vi "Edit_Raw_DF_Header.vi"(0 "Selected files":path[](array[path])) -> ()   [LabVIEW 2021]
uses:
  Controls/File_Selector_Type.ctl
  <vilib>/Utility/error.llb/whitespace.ctl
panel:
  out "All Metadata Names":string[](array[string])
  out "New Metadata":string[](array[string])
  out "Orig Full Metadata":string[][](array[string])
  out "Meta data changed?":bool[](array[boolean])
  out "Orig Metadata Values":string[](array[string])
  out "Number of Instuments":i32
  in  "Instrument Index":i32
  in  "MetaData to change":string[][](table)
  out "Cells to Change":i32[][](array[numeric])
  out "Original Values":string[][](array[string])
  in  "Analysis Info Cluster Setup to Edit":string[][](table)
  in  "Variable names to add by hand":string[](array[string])
  in  "Variable values to add by hand":string[](array[string])
  out "No of Unfound files":i32
  out "Unfound Files":path[](array[path])
  out "File Number":i32
  out "Current case":string
  out "Currently Editting":path
  out "Summary values":string[](array[string])
  in  "New Variable values":string[](array[string])
  in  "Setup Information":i32[](listbox)
  in  "Variable names to Edit":string[](array[string])
  in  "OK":bool
  out "No of Files":i32
  in  "Previous Choice":path
  in  "Search String":string
  in  "At Dialog Prompt for Editting Raw data files":T1
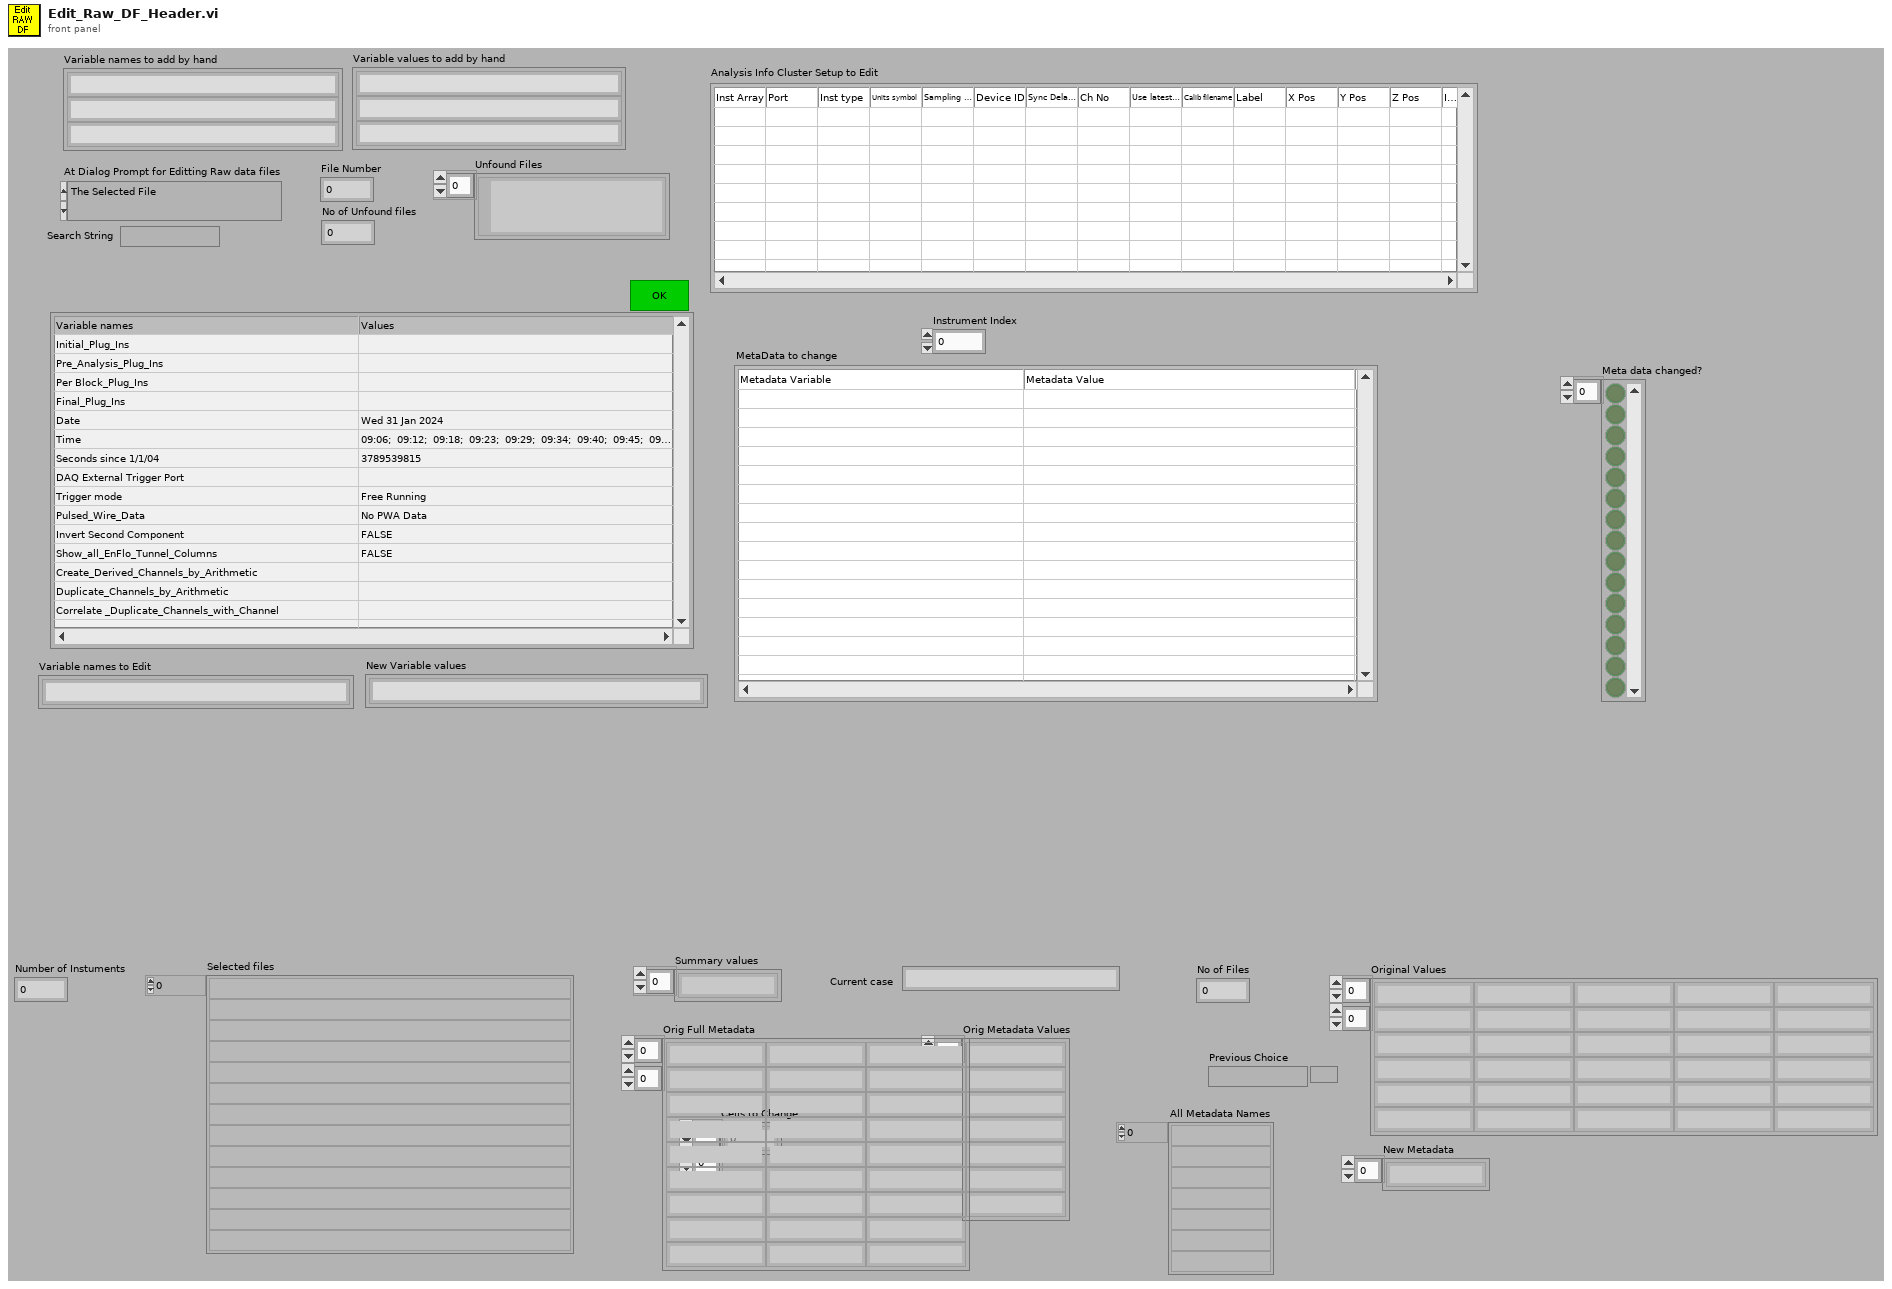
[diagram p1: front panel]
types:
  T1 = typedef "File_Selector_Type.ctl" = enum16{"The Selected File", "The Selected Folder", "Files containing the search string in the selected folder", "All files listed in selected file"}
  T2 = typedef "whitespace.ctl" = u16
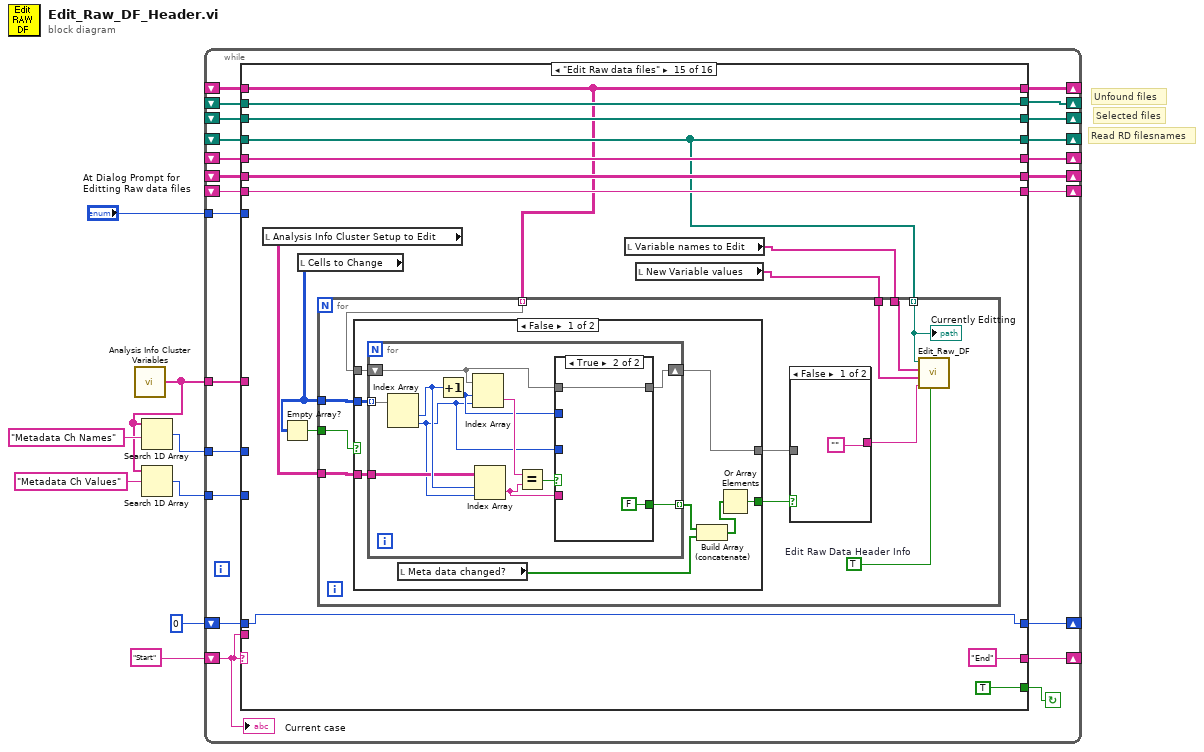
[diagram p0: block diagram]
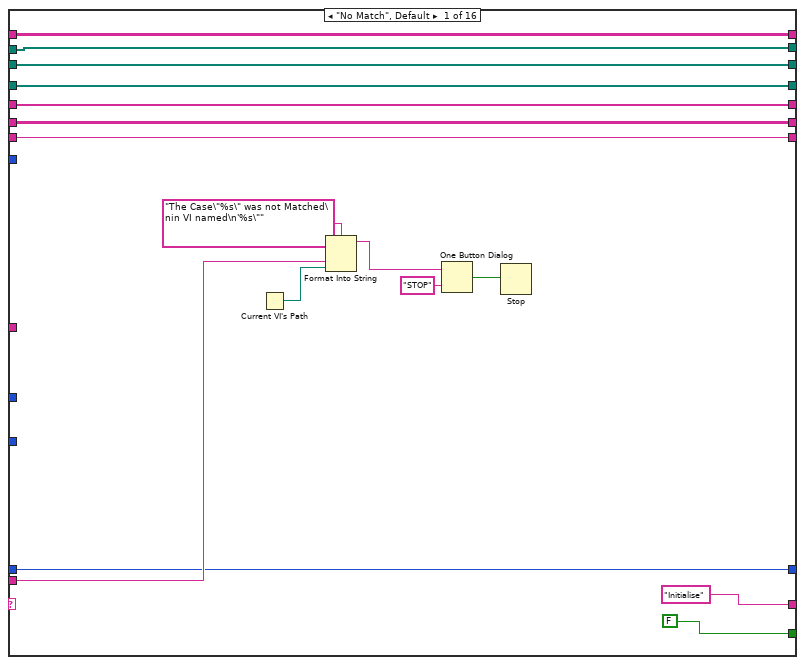
[diagram p2: hidden frame]
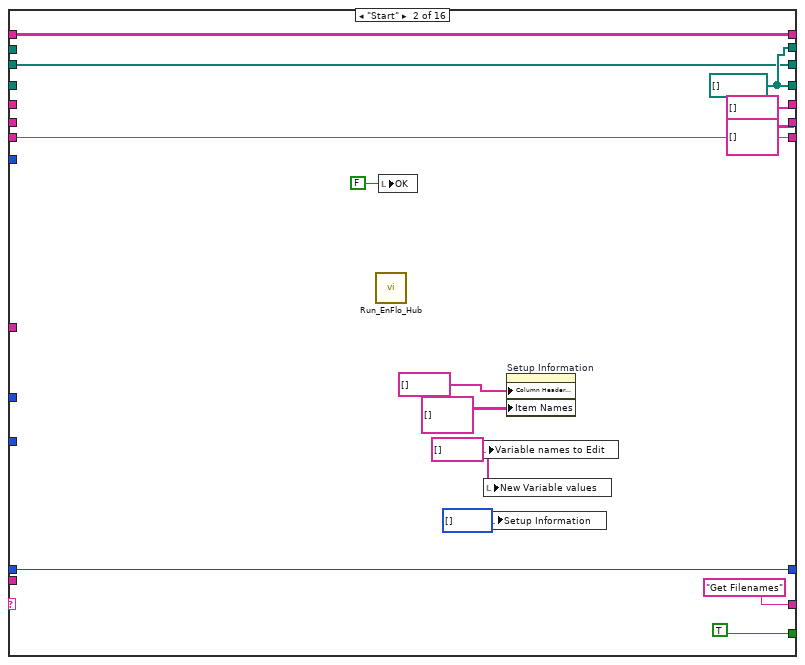
[diagram p3: hidden frame]
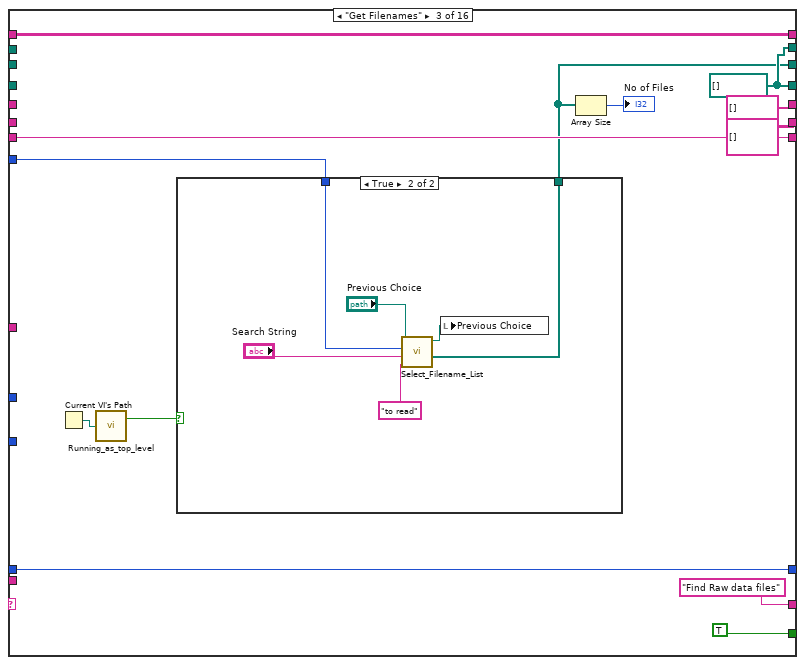
[diagram p4: hidden frame]
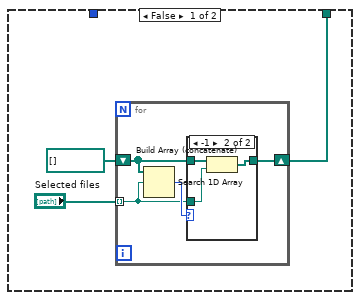
[diagram p5: hidden frame]
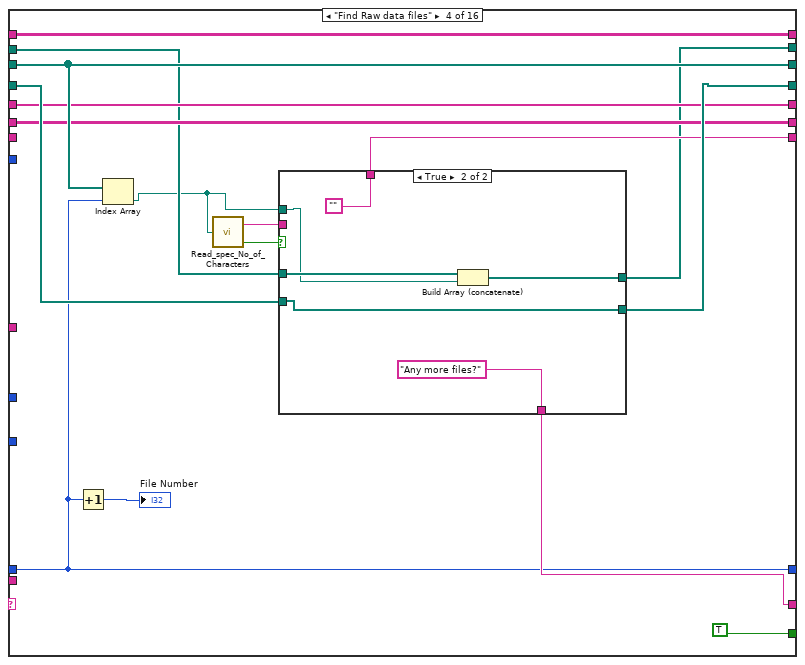
[diagram p7: hidden frame]
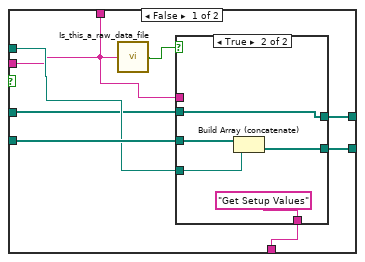
[diagram p8: hidden frame]
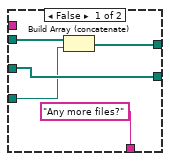
[diagram p9: hidden frame]
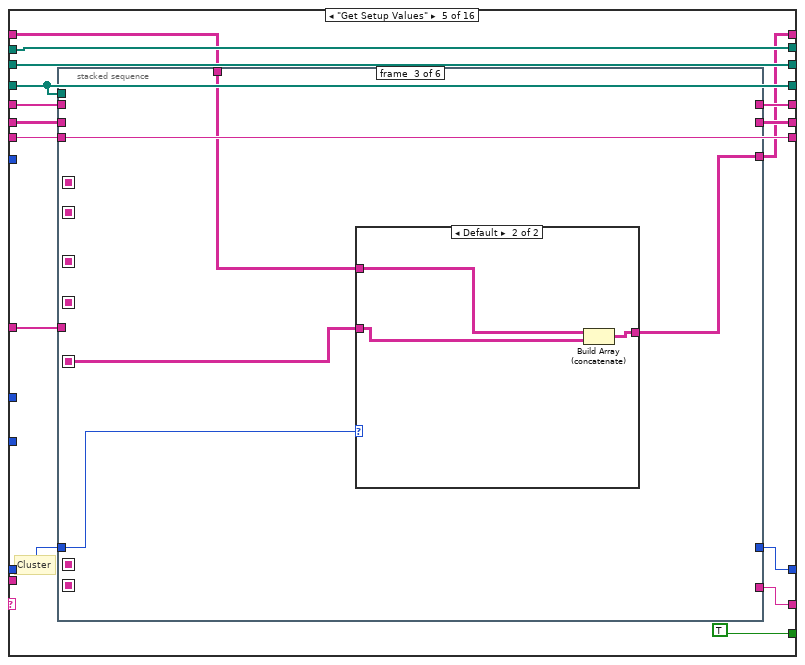
[diagram p10: hidden frame]
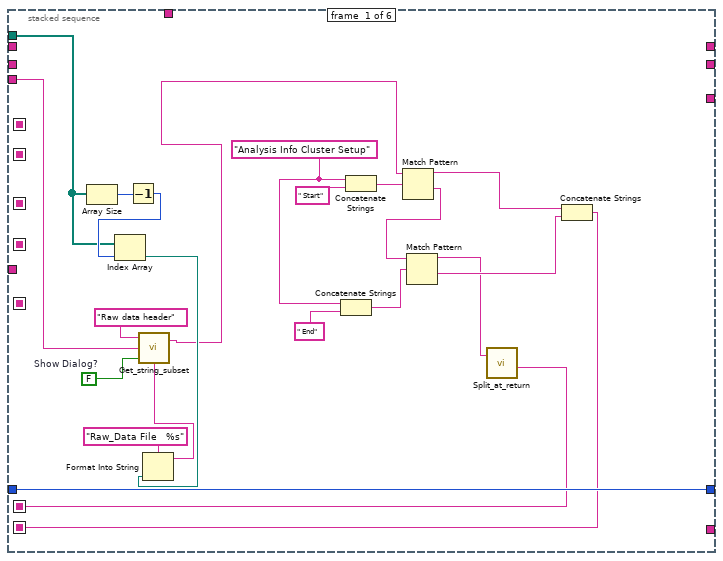
[diagram p11: hidden frame]
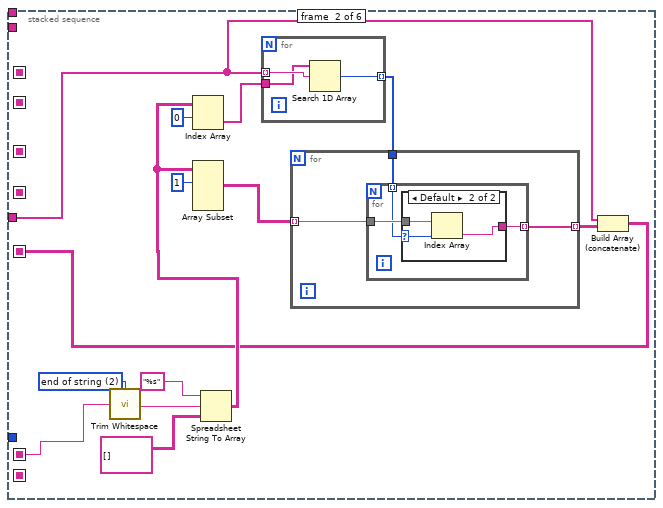
[diagram p12: hidden frame]
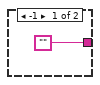
[diagram p13: hidden frame]
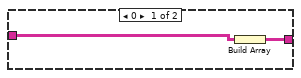
[diagram p14: hidden frame]
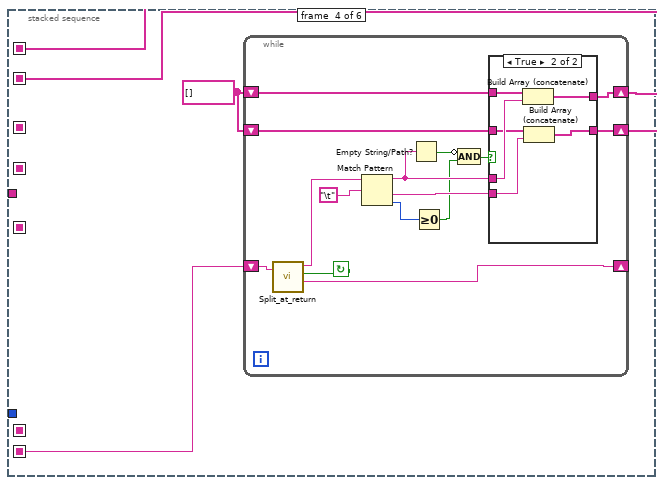
[diagram p15: hidden frame]
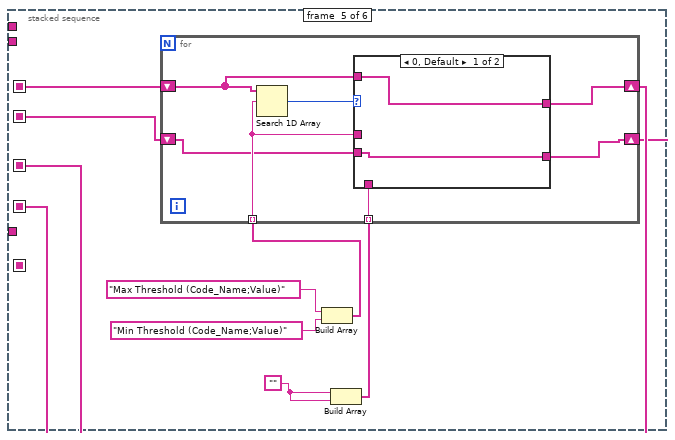
[diagram p17: hidden frame]
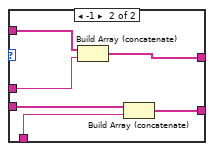
[diagram p18: hidden frame]
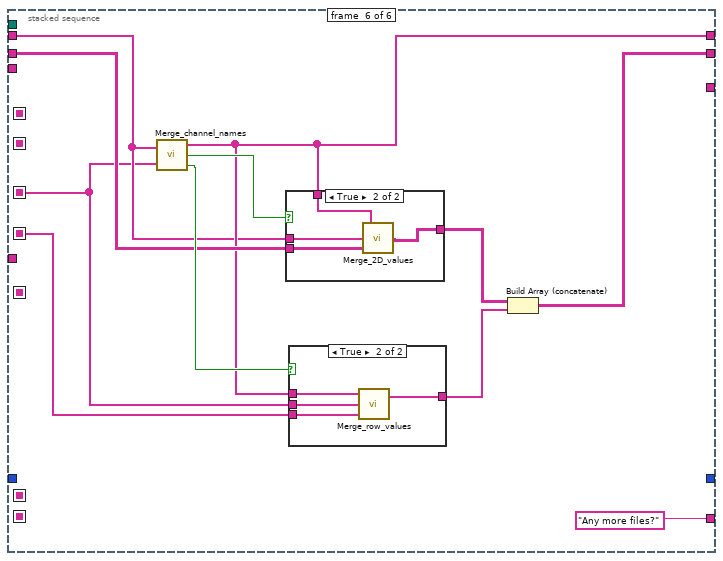
[diagram p19: hidden frame]
diagram:
  # "Selected files"
  # "Unfound files"
  # "Read RD filesnames"
  n1 = call "Analysis Info Cluster Variables.vi"() -> ("Array"=w3:string[])
  n2 = Search 1D Array(1D array=w3, element="Metadata Ch Names") -> (index of element=w1:i32)  [unwired: 1 in]
  n3 = Search 1D Array(1D array=w3, element="Metadata Ch Values") -> (index of element=w2:i32)  [unwired: 1 in]
  n4 = while {
    shift-left: "Start" -> [w29]
    shift-right: [w30] -> _
    shift-right: [w27] -> _
    shift-left: _ -> [w28]
    tunnel: "At Dialog Prompt for Editting Raw data files" -> [w26]
    shift-right: [w17] -> _
    shift-left: 0 -> [w23]
    shift-right: [w25] -> _
    shift-left: _ -> [w24]
    shift-right: [w22] -> _
    shift-left: _ -> [w21]
    shift-right: [w19] -> _
    shift-left: _ -> [w20]
    shift-right: [w18] -> _
    shift-left: _ -> [w16]
    shift-right: [w14] -> _
    shift-left: _ -> [w15]
    shift-right: [w13] -> _
    shift-left: _ -> [w12]
    tunnel: w3 -> [w11]
    tunnel: w2 -> [w10]
    tunnel: w1 -> [w9]
    stop <- w31 continue-if-true
    n5 = case shown="\"Edit Raw data files\"" w29 {
      tunnel: [FALSE TRUE TRUE TRUE TRUE TRUE TRUE TRUE TRUE TRUE ("T button?") TRUE w481 w551 TRUE ("T button?") TRUE ("T button?") FALSE ("T button?")] -> w31
      tunnel: ["Initialise" "Get Filenames" "Find Raw data files" w100 w142 w283 w303 "Summarise Analysis Cluster" "Metadata Channels" "user to select variables" w435 "Shall I edit the data files?" w544 "Edit Raw data files" ("f") "End" "End"] -> w30
      tunnel: w29 -> [w42 _ _ _ _ _ _ _ _ _ _ _ _ _ _ _]
      tunnel: w28 -> [w39 w49 _ w104 w145 w290 w309 w337 w365 w402 w441 w501 w560 w588 w634 w690]
      tunnel: [w39 w49 w63 w104 w145 w290 w309 w337 w365 w402 w441 w501 w560 w588 w634 w690] -> w27
      tunnel: w26 -> [_ _ w73 _ _ _ _ _ _ _ _ _ _ _ _ _]
      tunnel: w24 -> [w38 _ _ w106 w135 w282 w302 w334 w362 w401 w440 w498 w555 w587 w629 w684]
      tunnel: [w38 w50 w66 w105 w135 w282 w302 w334 w362 w401 w440 w498 w555 w587 w629 w684] -> w25
      tunnel: w23 -> [w34 w56 w67 w99 w144 w288 w308 w336 w364 w393 w434 w500 w556 w563 w630 w685]
      tunnel: [w37 string[] [] ("Merged Channels") string[] [] ("Merged Channels") w103 w140 w278 w297 w330 w359 w400 w436 w489 w557 w586 w631 w687] -> w22
      tunnel: w21 -> [w37 _ _ w103 w137 w278 w298 w330 w359 w400 w436 w489 w557 w586 w631 w687]
      tunnel: w20 -> [w36 _ _ w102 w139 w289 w294 w332 w360 w399 w438 w496 w558 w585 w632 w688]
      tunnel: [w36 string[][] [] string[][] [] w102 w138 w289 w293 w332 w360 w399 w438 w496 w558 w585 w632 w688] -> w19
      tunnel: [w35 w59 w70 w101 w141 w281 w301 w333 w361 w398 w439 w497 w559 w584 w633 w689] -> w18
      tunnel: [w34 w56 w67 w99 w143 w287 w307 w335 w363 w393 w434 w499 w556 w563 w630 w685] -> w17
      tunnel: w16 -> [w35 w59 w70 _ w141 w281 w301 w333 w361 w398 w439 w497 w559 w584 w633 w689]
      tunnel: w15 -> [w33 _ _ w98 w136 w279 w299 w323 w357 w403 w433 w490 w550 w583 w628 w680]
      tunnel: [w33 w50 w66 w97 w136 w279 w299 w323 w357 w403 w433 w490 w550 w583 w628 w680] -> w14
      tunnel: [w32 w48 w62 w92 w134 w277 w292 w321 w353 w396 w432 w482 w549 w565 w627 w679] -> w13
      tunnel: w12 -> [w32 w48 w62 w92 w133 w277 w292 w321 w353 w396 w432 w482 w549 w571 w627 w679]
      tunnel: w11 -> [_ _ _ _ w132 _ _ _ _ _ _ _ _ _ _ _]
      tunnel: w10 -> [_ _ _ _ _ _ _ _ _ w394 _ _ _ w567 _ _]
      tunnel: w9 -> [_ _ _ _ _ _ _ _ _ w395 _ _ _ w570 _ _]
      frame "No Match", Default {
        n6 = Current VI's Path() -> (path=w41:path)
        n7 = Format Into String(format string="The Case\"%s\" was not Matched\nin VI named\n'%s\"" ("Format String"), w42, w41) -> (resulting string=w45:string)  [unwired: 2 in, 1 out]
        n8 = One Button Dialog(message=w45, button name ("OK")="STOP") -> (true=w43:bool)
        n9 = Stop(stop? (T)=w43) -> ()
      }
      frame "Start" {
        w55 = string[] [] ("Variable names to Edit")
        w50 = path[] []
        n10 = call "Run_EnFlo_Hub.vi"() -> ()  [unwired: 1 in, 7 out]
        n11 = local write "OK"(FALSE ("OK")) -> ()
        n12 = local write "Variable names to Edit"(w55) -> ()
        n13 = local write "New Variable values"(w55) -> ()
        n14 = local write "Setup Information"(i32[] [] ("Setup Information")) -> ()
        n15 = property on="Setup Information" class="MCListbox (strict)"("Column Header Strings[]"=string[] [] ("Column Header Strings"), "Item Names"=string[][] []) -> ()  [unwired: 2 in, 2 out]
      }
      frame "Get Filenames" {
        w66 = path[] []
        n16 = Current VI's Path() -> (path=w65:path)
        n17 = call "Running_as_top_level.vi"("Vi path name"=w65) -> ("Top Level"=w64:bool)  [unwired: 1 out]
        n18 = case shown="True" w64 {
          tunnel: w73 -> [_ w91]
          tunnel: [w75 w86] -> w63
          frame False {
            n19 = for {
              shift-right: [w78] -> w75
              shift-left: path[] [] -> [w79]
              tunnel: "Selected files" -> [w80] mode=indexing
              n20 = Search 1D Array(1D array=w79, element=w80) -> (index of element=w81:i32)  [unwired: 1 in]
              n21 = case shown="-1" w81 {
                tunnel: w80 -> [_ w85]
                tunnel: w79 -> [w82 w84]
                tunnel: [w82 w83] -> w78
                frame Default {
                }
                frame -1 {
                  n22 = Build Array (concatenate)(w84, w85) -> (w83:path[])
                }
              }
            }
          }
          frame True {
            n23 = call "Select_Filename_List.vi"("File Type"="to read", "Search String"="Search String", "At Dialog Prompt Post Process"=w91, "Previous Choice"="Previous Choice") -> ("Selected files"=w86:path[], "Choosen path"=w87:path)  [unwired: 1 in, 2 out]
            n24 = local write "Previous Choice"(w87) -> ()
          }
        }
        n25 = Array Size(array=w63) -> (size(s)=→"No of Files":i32)
      }
      frame "Find Raw data files" {
        n26 = Increment(x=w99) -> (x+1=→"File Number":i32)
        n27 = Index Array(array=w104, index=w99) -> (element=w96:path)
        n28 = call "Read_spec_No_of_Characters.vi"("Filename"=w96) -> ("character string"=w94:string, "Error?"=w95:bool)
        n29 = case shown="True" w95 {
          tunnel: w106 -> [w115 w131]
          tunnel: [w114 w131] -> w105
          tunnel: w96 -> [w112 w127]
          tunnel: [w108 ""] -> w101
          tunnel: [w111 "Any more files?"] -> w100
          tunnel: w98 -> [w110 w128]
          tunnel: [w109 w126] -> w97
          tunnel: w94 -> [w108 _]
          frame False {
            n30 = call "Is_this_a_raw_data_file.vi"("character string"=w108) -> ("Raw Dat File?"=w113:bool)  [unwired: 2 out]
            n31 = case shown="True" w113 {
              tunnel: w115 -> [w120 w125]
              tunnel: w112 -> [w116 w124]
              tunnel: [w120 w123] -> w114
              tunnel: w108 -> [_ _]
              tunnel: ["Any more files?" "Get Setup Values"] -> w111
              tunnel: w110 -> [w118 w121]
              tunnel: [w117 w121] -> w109
              frame False {
                n32 = Build Array (concatenate)(w118, w116) -> (w117:path[])
              }
              frame True {
                n33 = Build Array (concatenate)(w125, w124) -> (w123:path[])
              }
            }
          }
          frame True {
            n34 = Build Array (concatenate)(w128, w127) -> (w126:path[])
          }
        }
      }
      frame "Get Setup Values" {
        # "Cluster"
        n35 = stacked-sequence {
          seq-local: [_ _ _ w207 _ _] -> [_ _ _ _ w240 _]
          seq-local: [_ _ _ w206 _ _] -> [_ _ _ _ w236 _]
          seq-local: [_ _ _ _ w233 _] -> [_ _ _ _ _ w257]
          seq-local: [_ _ _ _ w232 _] -> [_ _ _ _ _ w256]
          seq-local: [w149 _ _ _ _ _] -> [_ _ _ w205 _ _]
          seq-local: [w147 _ _ _ _ _] -> [_ w170 _ _ _ _]
          seq-local: [_ w172 _ _ _ _] -> [_ _ w196 _ _ _]
          tunnel: w144 -> [w165 _ w199 _ _ _]
          tunnel: [w165 _ _ _ _ _] -> w143
          tunnel: [_ _ _ _ _ "Any more files?"] -> w142
          tunnel: w141 -> [w166 _ _ _ _ _]
          tunnel: w137 -> [_ _ _ _ _ w258]
          tunnel: [_ _ _ _ _ w260] -> w140
          tunnel: w139 -> [_ _ _ _ _ w264]
          tunnel: [_ _ _ _ _ w261] -> w138
          tunnel: w135 -> [w160 _ _ _ _ _]
          tunnel: [_ _ w198 _ _ _] -> w134
          tunnel: w133 -> [_ _ w197 _ _ _]
          tunnel: w132 -> [_ w173 _ _ _ _]
          frame #0 {
            w155 = "Analysis Info Cluster Setup"
            w168 = FALSE  # Show Dialog?
            n36 = Array Size(array=w160) -> (size(s)=w162:i32)
            n37 = Decrement(x=w162) -> (x-1=w161:i32)
            n38 = Index Array(array=w160, index=w161) -> (element=w159:path)
            n39 = Format Into String(format string="Raw_Data File   %s", w159) -> (resulting string=w163:string)  [unwired: 2 in, 1 out]
            n40 = call "Get_string_subset.vi"("String Name"=w163, "Show Dialog?"=w168, "String to split"=w166, "File Label"="Raw data header") -> ("Output string"=w154:string)  [unwired: 1 out]
            n41 = Concatenate Strings(w155, " End") -> (w152:string)
            n42 = Concatenate Strings(w155, " Start") -> (w158:string)
            n43 = Match Pattern(string=w154, regular expression=w158) -> (before substring=w151:string, after substring=w153:string)  [unwired: 3 out]
            n44 = Match Pattern(string=w153, regular expression=w152) -> (before substring=w148:string, after substring=w150:string)  [unwired: 3 out]
            n45 = call "Split_at_return.vi"("String"=w148) -> ("after substring"=w147:string)  [unwired: 1 in, 3 out]
            n46 = Concatenate Strings(w151, w150) -> (w149:string)
          }
          frame #1 {
            w171 = T2 2 items=["both", "start of string", "end of string"] ("location (both)")
            n47 = call <vilib>:"Trim Whitespace.vi"("string"=w170, "location (both)"=w171) -> ("trimmed string"=w169:string)
            n48 = Spreadsheet String To Array(format string="%s", spreadsheet string=w169, array type (2D Dbl)=string[][] []) -> (array=w178:string[][])  [unwired: 1 in]
            n49 = Index Array(array=w178, index (row)=0) -> (element=w179:string[])  [unwired: 1 in]
            n50 = Array Subset(array=w178, index (row)=1 ("index")) -> (w176:string[][])  [unwired: 3 in]
            n51 = for {
              tunnel: w173 -> [w195] mode=indexing
              tunnel: w179 -> [w194]
              tunnel: [w193] -> w175 mode=indexing
              n52 = Search 1D Array(1D array=w194, element=w195) -> (index of element=w193:i32)  [unwired: 1 in]
            }
            n53 = for {
              tunnel: w176 -> [w185] mode=indexing
              tunnel: w175 -> [w184]
              tunnel: [w183] -> w174 mode=indexing
              n54 = for {
                tunnel: w185 -> [w188]
                tunnel: w184 -> [w187] mode=indexing
                tunnel: [w186] -> w183 mode=indexing
                n55 = case shown="Default" w187 {
                  selector: w187 -> [_ w191]
                  tunnel: w188 -> [_ w192]
                  tunnel: ["" w190] -> w186
                  frame -1 {
                  }
                  frame Default {
                    n56 = Index Array(array=w192, index=w191) -> (element=w190:string)
                  }
                }
              }
            }
            n57 = Build Array (concatenate)(w173, w174) -> (w172:string[][])
          }
          frame #2 {
            n58 = case shown="Default" w199 {
              tunnel: w196 -> [w201 w203]
              tunnel: [w200 w202] -> w198
              tunnel: w197 -> [_ w204]
              frame 0 {
                n59 = Build Array(w201) -> (w200:string[][][])
              }
              frame Default {
                n60 = Build Array (concatenate)(w204, w203) -> (w202:string[][][])
              }
            }
          }
          frame #3 {
            w208 = string[] []
            n61 = while {
              shift-right: [w222] -> _
              shift-left: w205 -> [w223]
              shift-right: [w216] -> w207
              shift-left: w208 -> [w217]
              shift-right: [w214] -> w206
              shift-left: w208 -> [w215]
              stop <- w221 continue-if-true
              n62 = call "Split_at_return.vi"("String"=w223) -> ("before substring"=w219:string, "Matched?"=w221:bool, "after substring"=w222:string)  [unwired: 1 in, 1 out]
              n63 = Match Pattern(string=w219, regular expression="\t") -> (before substring=w212:string, after substring=w213:string, offset past match=w218:i32)  [unwired: 2 out]
              n64 = Empty String/Path?(string/path=w212) -> (empty?=w211:bool)
              n65 = Greater Or Equal To 0?(x=w218) -> (x >= 0?=w209:bool)
              n66 = Compound Arithmetic op=AND(invert w211, w209) -> (w210:bool)
              n67 = case shown="True" w210 {
                tunnel: w217 -> [w225 w231]
                tunnel: w212 -> [_ w230]
                tunnel: [w225 w229] -> w216
                tunnel: w215 -> [w224 w228]
                tunnel: [w224 w227] -> w214
                tunnel: w213 -> [_ w226]
                frame False {
                }
                frame True {
                  n68 = Build Array (concatenate)(w231, w230) -> (w229:string[])
                  n69 = Build Array (concatenate)(w228, w226) -> (w227:string[])
                }
              }
            }
          }
          frame #4 {
            w234 = ""
            n70 = Build Array("Max Threshold (Code_Name;Value)", "Min Threshold (Code_Name;Value)") -> (w237:string[])
            n71 = Build Array(w234, w234) -> (w235:string[])
            n72 = for {
              shift-right: [w244] -> w233
              shift-left: w240 -> [w246]
              tunnel: w237 -> [w245] mode=indexing
              shift-right: [w241] -> w232
              shift-left: w236 -> [w243]
              tunnel: w235 -> [w242] mode=indexing
              n73 = Search 1D Array(1D array=w246, element=w245) -> (index of element=w247:i32)  [unwired: 1 in]
              n74 = case shown="0, Default" w247 {
                tunnel: w246 -> [w249 w255]
                tunnel: w245 -> [_ w254]
                tunnel: [w249 w253] -> w244
                tunnel: w243 -> [w248 w252]
                tunnel: w242 -> [_ w251]
                tunnel: [w248 w250] -> w241
                frame 0, Default {
                }
                frame -1 {
                  n75 = Build Array (concatenate)(w255, w254) -> (w253:string[])
                  n76 = Build Array (concatenate)(w252, w251) -> (w250:string[])
                }
              }
            }
          }
          frame #5 {
            n77 = call "Merge_channel_names.vi"("Preferred Channel array"=w258, "Channel array"=w257) -> ("Merged Channels"=w260:string[], "Preferred Channels Changed?"=w265:bool, "Channel Array Changed?"=w266:bool)
            n78 = case shown="True" w265 {
              tunnel: w264 -> [w272 w274]
              tunnel: w258 -> [_ w276]
              tunnel: [w272 w273] -> w263
              tunnel: w260 -> [_ w275]
              frame False {
              }
              frame True {
                n79 = call "Merge_2D_values.vi"("Values In"=w274, "Present Channels"=w276, "Desired Channels"=w275) -> ("Values Out"=w273:string[][])
              }
            }
            n80 = case shown="True" w266 {
              tunnel: [w267 w271] -> w262
              tunnel: w260 -> [_ w270]
              tunnel: w257 -> [_ w269]
              tunnel: w256 -> [w267 w268]
              frame False {
              }
              frame True {
                n81 = call "Merge_row_values.vi"("Present Row values"=w268, "Present Channels"=w269, "Desired Channels"=w270) -> ("Desired Row values"=w271:string[])  [unwired: 1 out]
              }
            }
            n82 = Build Array (concatenate)(w263, w262) -> (w261:string[][])
          }
        }
      }
      frame "Any more files?" {
        n83 = Increment(x=w288) -> (x+1=w287:i32)
        n84 = local read "No of Files"() -> (w286:i32)
        n85 = Less?(x=w287, y=w286) -> (x < y?=w285:bool)
        n86 = Select(t="Find Raw data files", s=w285, f="Add Skip Blocks Variable") -> (s? t:f=w283:string)
      }
      frame "Add Skip Blocks Variable" {
        w296 = "Skip_Block_Numbers_(eg 1;2;5;12)" ("Variable name")
        n87 = Increment(x=w308) -> (x+1=w307:i32)
        n88 = Search 1D Array(1D array=w298, element=w296) -> (index of element=w295:i32)  [unwired: 1 out]
        n89 = case shown="-1" w295 {
          tunnel: w298 -> [w312 w317]
          tunnel: w296 -> [_ w316]
          tunnel: [w312 w315] -> w297
          tunnel: w294 -> [w311 w314]
          tunnel: [w311 w313] -> w293
          frame 0, Default {
          }
          frame -1 {
            n90 = for {
              tunnel: w314 -> [w319] mode=indexing
              tunnel: [w318] -> w313 mode=indexing
              n91 = Build Array (concatenate)(w319, "") -> (w318:string[])
            }
            n92 = Build Array (concatenate)(w317, w316) -> (w315:string[])
          }
        }
        n93 = local read "No of Files"() -> (w306:i32)
        n94 = Less?(x=w307, y=w306) -> (x < y?=w305:bool)
        n95 = Select(t="Find Raw data files", s=w305, f="Summarise data") -> (s? t:f=w303:string)
      }
      frame "Summarise data" {
        n96 = Increment(x=w336) -> (x+1=w335:i32)
        n97 = Array Size(array=w330) -> (size(s)=w331:i32)
        n98 = for {
          N: w331 -> [_]
          tunnel: w332 -> [w346]
          tunnel: [w342] -> w329 mode=indexing
          i -> [w347]
          w343 = FALSE  # Average Numeric Values?
          n99 = Index Array(array=w346, index (col)=w347) -> (element=w345:string[])  [unwired: 1 in]
          n100 = call "Value_Occurence_Analysis.vi"("Average Numeric Values?"=w343, "Tolerance"=0.5, "String Array"=w345) -> ("Output String"=w342:string)  [unwired: 1 in, 2 out]
        }
        "Summary values" <- w329
        n101 = for {
          tunnel: w330 -> [w340] mode=indexing
          tunnel: w329 -> [w341] mode=indexing
          tunnel: [w339] -> w325 mode=indexing
          n102 = Build Array(w340, w341) -> (w339:string[])
        }
        n103 = Array Size(array=w323) -> (size(s)=→"No of Unfound files":i32)
        n104 = Build Array("Variable names", "Values") -> (w324:string[])
        n105 = property on="Setup Information" class="MCListbox (strict)"("Column Header Strings[]"=w324, "Item Names"=w325) -> ()  [unwired: 2 in, 2 out]
        "Unfound Files" <- w323
      }
      frame "Summarise Analysis Cluster" {
        n106 = Array Size(array=w353) -> (size(s)=w356:i32[])
        n107 = Index Array(array=w356) -> (element #2=w355:i32, element #3=w354:i32)  [unwired: 3 in, 1 out]
        "Number of Instuments" <- w355
        n108 = Increment(x=w364) -> (x+1=w363:i32)
        n109 = for {
          N: w355 -> [_]
          tunnel: w353 -> [w369]
          tunnel: [w370] -> w351 mode=indexing
          tunnel: w354 -> [w367]
          i -> [w368]
          n110 = for {
            N: w367 -> [_]
            tunnel: [w372] -> w370 mode=indexing
            tunnel: w369 -> [w375]
            tunnel: w368 -> [w374]
            i -> [w373]
            n111 = Index Array(array=w375, index (dim 1)=w374, index (dim 2)=w373) -> (element=w371:string[])  [unwired: 1 in]
            n112 = call "Value_Occurence_Analysis.vi"("Average Numeric Values?"=FALSE, "Tolerance"=0.5, "String Array"=w371) -> ("Output String"=w372:string)  [unwired: 1 in, 2 out]
          }
        }
        n113 = Array Subset(array=w351, index (row)=1 ("index")) -> (w349:string[][])  [unwired: 3 in]
        "Original Values" <- w349
        n114 = local write "Analysis Info Cluster Setup to Edit"(w349) -> ()
        n115 = Index Array(array=w351, index (row)=0) -> (element=w348:string[])  [unwired: 1 in]
        n116 = property on="Analysis Info Cluster Setup to Edit" class="Tbl (strict)"("Column Headers[]"=w348) -> ()  [unwired: 2 in, 2 out]
      }
      frame "Metadata Channels" {
        n117 = local read "Number of Instuments"() -> (w383:i32)
        n118 = Array Subset(array=w396, index (dim 1)=1 ("index")) -> (w390:string[][][])  [unwired: 5 in]
        n119 = Greater?(x=w383, y="Instrument Index") -> (0:w382:bool)
        n120 = case shown="False" w382 {
          tunnel: [w404 w405] -> w381
          tunnel: "Instrument Index" -> [w404 _]
          frame False {
          }
          frame True {
            w405 = 0 ("Instrument Index")
            n121 = local write "Instrument Index"(w405) -> ()
          }
        }
        n122 = Index Array(array=w390, index (dim 1)=w381, index (dim 2)=w395) -> (element=w388:string[])  [unwired: 1 in]
        n123 = Index Array(array=w390, index (dim 1)=w381, index (dim 2)=w394) -> (element=w387:string[])  [unwired: 1 in]
        n124 = for {
          tunnel: w388 -> [w430] mode=indexing
          tunnel: [w429] -> w389 mode=concatenating
          n125 = call "String_2_String_Array.vi"("delimiter (;)"=";", "String"=w430) -> ("String Array"=w429:string[])  [unwired: 9 in]
        }
        n126 = call "Analyse_string_array.vi"("String array"=w389) -> ("Unique strings"=w385:string[])  [unwired: 1 in, 1 out]
        "All Metadata Names" <- w385
        n127 = for {
          tunnel: w388 -> [w418] mode=indexing
          tunnel: w387 -> [w416] mode=indexing
          tunnel: w385 -> [w415]
          tunnel: [w412] -> w386 mode=indexing
          n128 = call "String_2_String_Array.vi"("delimiter (;)"=";", "String"=w416) -> ("String Array"=w413:string[])  [unwired: 9 in]
          n129 = call "String_2_String_Array.vi"("delimiter (;)"=";", "String"=w418) -> ("String Array"=w414:string[])  [unwired: 9 in]
          n130 = for {
            tunnel: w415 -> [w424] mode=indexing
            tunnel: w414 -> [w423]
            tunnel: w413 -> [w421]
            tunnel: [w420] -> w412 mode=indexing
            n131 = Search 1D Array(1D array=w423, element=w424) -> (index of element=w422:i32)  [unwired: 1 in]
            n132 = case shown="-1" w422 {
              selector: w422 -> [w426 _]
              tunnel: w421 -> [w427 _]
              tunnel: [w425 ""] -> w420
              frame 0, Default {
                n133 = Index Array(array=w427, index=w426) -> (element=w425:string)
              }
              frame -1 {
              }
            }
          }
        }
        n134 = Transpose 2D Array(2D array=w386) -> (transposed array=w378:string[][])
        "Orig Full Metadata" <- w378
        n135 = for {
          tunnel: w378 -> [w409] mode=indexing
          tunnel: w385 -> [w408] mode=indexing
          tunnel: [w407] -> w384 mode=indexing
          tunnel: [w406] -> w379 mode=indexing
          n136 = call "Value_Occurence_Analysis.vi"("Average Numeric Values?"=FALSE, "Tolerance"=0.5, "String Array"=w409) -> ("Output String"=w406:string)  [unwired: 1 in, 2 out]
          n137 = Build Array(w408, w406) -> (w407:string[])
        }
        "Orig Metadata Values" <- w379
        n138 = local write "MetaData to change"(w384) -> ()
      }
      frame "user to select variables" {
        n139 = event shown="[0] \"Setup Information\": Value Change" {
          selector: _ -> [_ _]
          dyn-events: _ -> [_ _]
          timeout: _ -> [_ _]
          tunnel: w436 -> [w450 _]
          tunnel: ["user to select variables" "Any files to edit?"] -> w435
          event "Setup Information": Value Change {
            n140 = event-data() -> ("NewVal"=w451:i32[])  [unwired: 6 out]
            n141 = local read "Summary values"() -> (w449:string[])
            n142 = for {
              tunnel: w451 -> [w457] mode=indexing
              tunnel: w450 -> [w460]
              tunnel: "Variable names to Edit" -> [w459]
              tunnel: [w458] -> w443 mode=indexing
              tunnel: w449 -> [w456]
              tunnel: [w455] -> w448 mode=indexing
              tunnel: "New Variable values" -> [w453]
              tunnel: [w452] -> w445
              i -> [w452]
              n143 = Index Array(array=w460, index=w457) -> (element=w458:string)
              n144 = Search 1D Array(1D array=w459, element=w458) -> (index of element=w454:i32)  [unwired: 1 out]
              n145 = case shown="-1" w454 {
                tunnel: w457 -> [_ w466]
                tunnel: w456 -> [_ w465]
                tunnel: [w461 w464] -> w455
                tunnel: w454 -> [w463 _]
                tunnel: w453 -> [w462 _]
                frame 0, Default {
                  n146 = Index Array(array=w462, index=w463) -> (element=w461:string)
                }
                frame -1 {
                  n147 = Index Array(array=w465, index=w466) -> (element=w464:string)
                }
              }
            }
            n148 = Increment(x=w445) -> (x+1=w444:i32)
            n149 = local write "New Variable values"(w448) -> ()
            n150 = local write "Variable names to Edit"(w443) -> ()
            n151 = property on="Variable names to Edit" class="Arr (strict)"("Number of Rows"=w444) -> ()  [unwired: 2 in, 2 out]
            n152 = property on="New Variable values" class="Arr (strict)"("Number of Rows"=w444) -> ()  [unwired: 2 in, 2 out]
          }
          event "OK": Value Change {
            n153 = event-data() -> ()  [unwired: 7 out]
          }
        }
      }
      frame "Any files to edit?" {
        w492 = string[] []
        n154 = local read "New Variable values"() -> (w488:string[])
        n155 = Increment(x=w500) -> (x+1=w499:i32)
        n156 = local read "Summary values"() -> (w493:string[])
        n157 = local read "Original Values"() -> (w479:string[][])
        n158 = local read "Variable names to Edit"() -> (w485:string[])
        n159 = Build Array (concatenate)("Variable values to add by hand", w488) -> (w486:string[])
        n160 = for {
          tunnel: "Analysis Info Cluster Setup to Edit" -> [w506] mode=indexing
          tunnel: w479 -> [w505] mode=indexing
          shift-right: [w502] -> w477
          shift-left: i32[][] [] -> [w503]
          i -> [w504]
          n161 = for {
            tunnel: w506 -> [w513] mode=indexing
            tunnel: w505 -> [w512] mode=indexing
            tunnel: w504 -> [w511]
            shift-right: [w508] -> w502
            shift-left: w503 -> [w507]
            i -> [w510]
            n162 = Equal?(x=w513, y=w512) -> (x = y?=w509:bool)
            n163 = case shown="False" w509 {
              tunnel: w511 -> [w518 _]
              tunnel: w510 -> [w517 _]
              tunnel: [w515 w519] -> w508
              tunnel: w507 -> [w514 w519]
              frame False {
                n164 = Build Array(w518, w517) -> (w516:i32[])
                n165 = Build Array (concatenate)(w516, w514) -> (w515:i32[][])
              }
              frame True {
              }
            }
          }
        }
        "Cells to Change" <- w477
        n166 = Build Array (concatenate)("Variable names to add by hand", w485) -> (w483:string[])
        n167 = for {
          tunnel: "Setup Information" -> [w522]
          tunnel: w493 -> [w535]
          tunnel: w486 -> [w529] mode=indexing
          shift-right: [w532] -> w491
          shift-left: w492 -> [w533]
          shift-right: [w530] -> w475
          shift-left: w492 -> [w531]
          tunnel: w483 -> [w527] mode=indexing
          tunnel: w489 -> [w528]
          i -> [w521]
          n168 = Index Array(array=w522, index=w521) -> (element=w520:i32)
          n169 = Index Array(array=w528, index=w520) -> (element=w526:string)
          n170 = Index Array(array=w535, index=w520) -> (element=w534:string)
          n171 = Equal?(x=w534, y=w529) -> (x = y?=w525:bool)
          n172 = Equal?(x=w527, y=w526) -> (x = y?=w524:bool)
          n173 = And(x=w524, y=w525) -> (x .and. y?=w523:bool)
          n174 = case shown="False" w523 {
            tunnel: w533 -> [w541 w543]
            tunnel: [w540 w543] -> w532
            tunnel: w531 -> [w539 w542]
            tunnel: [w538 w542] -> w530
            tunnel: w529 -> [w537 _]
            tunnel: w527 -> [w536 _]
            frame False {
              n175 = Build Array (concatenate)(w539, w537) -> (w538:string[])
              n176 = Build Array (concatenate)(w541, w536) -> (w540:string[])
            }
            frame True {
            }
          }
        }
        n177 = local write "Variable names to Edit"(w491) -> ()
        n178 = local read "Orig Metadata Values"() -> (w470:string[])
        n179 = Empty Array?(array=w477) -> (empty?=w476:bool)
        n180 = Index Array(array="MetaData to change", index (col)=1 ("disabled index (col)")) -> (element=w471:string[])  [unwired: 1 in]
        "New Metadata" <- w471
        n181 = local write "New Variable values"(w475) -> ()
        n182 = Empty Array?(array=w475) -> (empty?=w474:bool)
        n183 = Not Equal?(x=w471, y=w470) -> (x != y?=w469:bool[])
        "Meta data changed?" <- w469
        n184 = Or Array Elements(Boolean array=w469) -> (logical OR=w468:bool)
        n185 = Compound Arithmetic op=OR(w468, invert w474, invert w476) -> (w481:bool)
      }
      frame "Shall I edit the data files?" {
        n186 = Array Size(array=w555) -> (size(s)=w554:i32)
        n187 = local read "Meta data changed?"() -> (w548:bool[])
        n188 = Format Into String(format string="Do you want to edit these raw data header values in %d Raw Data Files?" ("message"), w554) -> (resulting string=w552:string)  [unwired: 2 in, 1 out]
        n189 = Or Array Elements(Boolean array=w548) -> (logical OR=w547:bool)
        n190 = Two Button Dialog(message=w552) -> (T button?=w551:bool)  [unwired: 2 out]
        n191 = Select(t="Update metadata", s=w547, f="Edit Raw data files") -> (s? t:f=w544:string)
        n192 = property on="Currently Editting" class="Path"("Visible"=w551) -> ()  [unwired: 2 in, 2 out]
      }
      frame "Update metadata" {
        n193 = local read "Orig Full Metadata"() -> (w581:string[][])
        n194 = local read "Instrument Index"() -> (w569:i32)
        n195 = local read "Meta data changed?"() -> (w582:bool[])
        n196 = local read "All Metadata Names"() -> (w576:string[])
        n197 = local read "New Metadata"() -> (w578:string[])
        n198 = Array Size(array=w581) -> (size(s)=w580:i32[])
        n199 = Increment(x=w569) -> (x+1=w561:i32)
        n200 = Index Array(array=w580, index=1) -> (element=w579:i32)
        n201 = for {
          tunnel: w582 -> [w615] mode=indexing
          tunnel: [w614] -> w577 mode=indexing
          tunnel: w581 -> [w613] mode=indexing
          tunnel: w579 -> [w612]
          tunnel: w578 -> [w611] mode=indexing
          n202 = case shown="True" w615 {
            tunnel: [w616 w617] -> w614
            tunnel: w613 -> [w616 _]
            tunnel: w612 -> [_ w619]
            tunnel: w611 -> [_ w618]
            frame False {
            }
            frame True {
              n203 = Initialize Array(w618, w619) -> (w617:string[])
            }
          }
        }
        n204 = for {
          shift-right: [w607] -> w568
          shift-left: "" -> [w610]
          tunnel: ";" ("delimiter (Tab)") -> [w609]
          tunnel: w576 -> [w606] mode=indexing
          n205 = call <vilib>:"Space Constant.vi"() -> ("String"=w608:string)
          n206 = Concatenate Strings(w610, w606, w609, w608) -> (w607:string)
        }
        n207 = Transpose 2D Array(2D array=w577) -> (transposed array=w575:string[][])
        n208 = for {
          tunnel: w575 -> [w598] mode=indexing
          tunnel: [w597] -> w566 mode=indexing
          n209 = for {
            shift-right: [w602] -> w597
            shift-left: "" -> [w605]
            tunnel: ";" ("delimiter (Tab)") -> [w604]
            tunnel: w598 -> [w601] mode=indexing
            n210 = call <vilib>:"Space Constant.vi"() -> ("String"=w603:string)
            n211 = Concatenate Strings(w605, w601, w604, w603) -> (w602:string)
          }
        }
        n212 = for {
          tunnel: w571 -> [w594] mode=indexing
          tunnel: w570 -> [w590]
          tunnel: w561 -> [w591]
          tunnel: w568 -> [w596]
          tunnel: w567 -> [w589]
          tunnel: w566 -> [w595] mode=indexing
          tunnel: [w593] -> w565 mode=indexing
          n213 = Replace Array Subset(array=w594, new element=w596, index (row)=w591, index (col)=w590) -> (w592:string[][])
          n214 = Replace Array Subset(array=w592, new element=w595, index (row)=w591, index (col)=w589) -> (w593:string[][])
        }
      }
      frame "Edit Raw data files" {
        n215 = local read "Analysis Info Cluster Setup to Edit"() -> (w626:string[][])
        n216 = local read "Cells to Change"() -> (w621:i32[][])
        n217 = Empty Array?(array=w621) -> (empty?=w620:bool)
        n218 = local read "Variable names to Edit"() -> (w625:string[])
        n219 = local read "New Variable values"() -> (w624:string[])
        n220 = for {
          tunnel: w627 -> [w644] mode=indexing
          tunnel: w621 -> [w636]
          tunnel: w626 -> [w645]
          tunnel: w625 -> [w641]
          tunnel: w624 -> [w640]
          tunnel: w629 -> [w637] mode=indexing
          tunnel: w620 -> [w635]
          w638 = TRUE  # Edit Raw Data Header Info
          n221 = case shown="False" w635 {
            tunnel: w645 -> [w653 _]
            tunnel: w644 -> [w652 w674]
            tunnel: [w651 w674] -> w643
            tunnel: [w650 TRUE] -> w642
            tunnel: w636 -> [w649 _]
            frame False {
              n222 = for {
                tunnel: w649 -> [w664] mode=indexing
                tunnel: w653 -> [w662]
                shift-right: [w660] -> w651
                shift-left: w652 -> [w659]
                tunnel: [w654] -> w648 mode=indexing
                n223 = Index Array(array=w664) -> (element #1=w663:i32, element #2=w657:i32)  [unwired: 2 in]
                n224 = Increment(x=w663) -> (x+1=w658:i32)
                n225 = Index Array(array=w659, index (row)=w658, index (col)=w657) -> (element=w661:string)
                n226 = Index Array(array=w662, index (row)=w663, index (col)=w657) -> (element=w656:string)
                n227 = Equal?(x=w661, y=w656) -> (x = y?=w655:bool)
                n228 = case shown="True" w655 {
                  tunnel: [w669 w672] -> w660
                  tunnel: w659 -> [w670 w672]
                  tunnel: w658 -> [w668 _]
                  tunnel: w657 -> [w667 _]
                  tunnel: w656 -> [w666 _]
                  tunnel: [TRUE FALSE] -> w654
                  frame False {
                    n229 = Replace Array Subset(array=w670, new element=w666, index (row)=w668, index (col)=w667) -> (w669:string[][])
                  }
                  frame True {
                  }
                }
              }
              n230 = local read "Meta data changed?"() -> (w646:bool[])
              n231 = Build Array (concatenate)(w648, w646) -> (w647:bool[])
              n232 = Or Array Elements(Boolean array=w647) -> (logical OR=w650:bool)
            }
            frame True {
            }
          }
          n233 = case shown="False" w642 {
            tunnel: w643 -> [_ w677]
            tunnel: ["" w676] -> w639
            frame False {
            }
            frame True {
              n234 = Array To Spreadsheet String(array=w677, 3:"%s" ("format string")) -> (spreadsheet string=w676:string)  [unwired: 1 in]
            }
          }
          n235 = call "Edit_Raw_DF.vi"("Edit Raw Data Header Info"=w638, "New Analysis Info Cluster Setup"=w639, "New Values In"=w640, "New Chs In"=w641, "Data filename"=w637) -> ()  [unwired: 1 in, 4 out]
          "Currently Editting" <- w637
        }
      }
      frame "End" {
        n236 = property on="Currently Editting" class="Path"("Visible"=FALSE) -> ()  [unwired: 2 in, 2 out]
        n237 = local write "OK"(FALSE ("OK")) -> ()
      }
    }
    "Current case" <- w29
  }
